vi "Timestamp with error IO.vi"(8 "error in (no error)":errorcluster) -> (0 "error out":errorcluster, 3 "current time":timestamp)   [LabVIEW 2013, in "Timing Lib.lvlib"]
doc: "Reentrant wrappe around get current time node with error IO for data flow."
uses:
  Timing Lib.lvlib
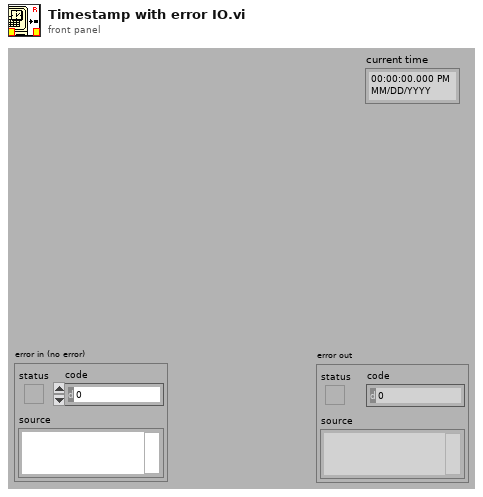
[diagram p1: front panel]
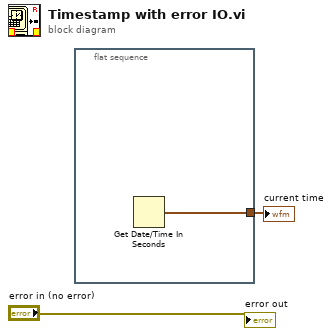
[diagram p0: block diagram]
diagram:
  n1 = flat-sequence {
    tunnel: [w3] -> w2
    frame #0 {
      n2 = Get Date/Time In Seconds() -> (seconds since 1Jan1904=w3:timestamp)
    }
  }
  "current time" <- w2
  "error out" <- "error in (no error)"
